vi "deadband sim.vi"(8 "Deadband (%)":dbl format="%.1f", 11 "requested pos. (%)":dbl format="%.2f") -> (1 "actual pos. (%)":dbl)   [LabVIEW 2010]
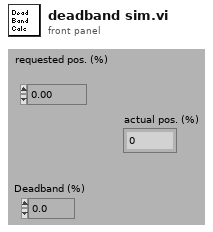
[diagram p1: front panel]
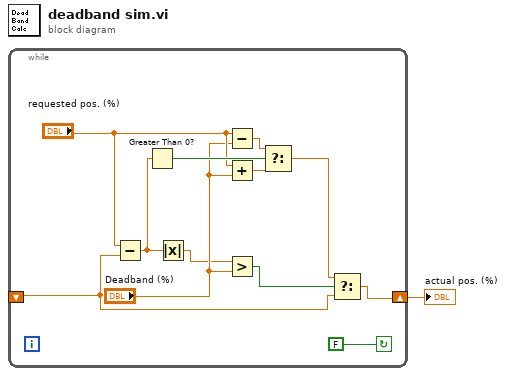
[diagram p0: block diagram]
diagram:
  n1 = while {
    shift-right: [w8] -> w1
    shift-left: _ -> [w5]
    stop <- FALSE continue-if-true
    n2 = Subtract(x="requested pos. (%)", y=w5) -> (x-y=w4:dbl)
    n3 = Greater Than 0?(x=w4) -> (x > 0?=w11:bool)
    n4 = Absolute Value(x=w4) -> (abs(x)=w3:dbl)
    n5 = Subtract(x="requested pos. (%)", y="Deadband (%)") -> (x-y=w12:dbl)
    n6 = Add(x="requested pos. (%)", y="Deadband (%)") -> (x+y=w10:dbl)
    n7 = Greater?(x=w3, y="Deadband (%)") -> (0:w2:bool)
    n8 = Select(t=w12, s=w11, f=w10) -> (s? t:f=w7:dbl)
    n9 = Select(t=w7, s=w2, f=w5) -> (s? t:f=w8:dbl)
  }
  "actual pos. (%)" <- w1
